vi "WritePathFile_Example.vi"(11 "Max Velocity M/S":dbl=3.2 format="%17.3f") -> (1 "PathPlannerTrajectory":T13 {"States"."TargetHolonomicRotation"."SIN" format="%13.4f"; "States"."TargetHolonomicRotation"."COS" format="%13.4f"; "States"."TargetHolonomicRotation"."VALUE" format="%13.4f"; "States"."Heading"."SIN" format="%13.4f"; "States"."Heading"."COS" format="%13.4f"; "States"."Heading"."VALUE" format="%13.4f"; "States"."PositionMeters"."Y" format="%14.3f"; "States"."PositionMeters"."X" format="%14.3f"}, 2 "Trajectory State\nCount":i32, 3 "TotalTImeSecs":dbl)   [LabVIEW 2019]
uses:
  <vilib>/Rock Robotics/WPI/ThirdParty/MJansen/PathPlanner/TypeDef/PathPlannerTrajectory.ctl
  <vilib>/Rock Robotics/WPI/ThirdParty/MJansen/PathPlanner/TypeDef/PathPlannerTrajectoryState.ctl
  <vilib>/Rock Robotics/WPI/ThirdParty/JAS_Junk/TrajLib/TypeDef/TRANSLATION2D.ctl
  <vilib>/Rock Robotics/WPI/ThirdParty/JAS_Junk/TrajLib/TypeDef/ROTATION2D.ctl
  <vilib>/Rock Robotics/WPI/ThirdParty/MJansen/PathPlanner/TypeDef/PathPlannerPathConstraints.ctl
  <vilib>/Rock Robotics/WPI/ThirdParty/MJansen/PathPlanner/TypeDef/PathPlannerPath.ctl
  <vilib>/Rock Robotics/WPI/ThirdParty/MJansen/PathPlanner/TypeDef/PathPlannerRotationTarget.ctl
  <vilib>/Rock Robotics/WPI/ThirdParty/MJansen/PathPlanner/TypeDef/PathPlannerConstraintsZone.ctl
  <vilib>/Rock Robotics/WPI/ThirdParty/MJansen/PathPlanner/TypeDef/PathPlannerEventMarker.ctl
  <vilib>/Rock Robotics/WPI/ThirdParty/MJansen/PathPlanner/TypeDef/PathPlannerCommandUtil.ctl
  <vilib>/Rock Robotics/WPI/ThirdParty/MJansen/PathPlanner/ENum/PathPlanner_CommandUtilType_ENUM.ctl
  <vilib>/Rock Robotics/WPI/ThirdParty/MJansen/PathPlanner/TypeDef/PathPlannerGoalEndState.ctl
  <vilib>/Rock Robotics/WPI/ThirdParty/MJansen/PathPlanner/TypeDef/PathPlannerPathPoint.ctl
  <vilib>/Rock Robotics/WPI/ThirdParty/JAS_Junk/TrajLib/Rotation2d_CreateAngle.vi
  <vilib>/Rock Robotics/WPI/ThirdParty/JAS_Junk/TrajLib/Translation2d_Create.vi
  <vilib>/Rock Robotics/WPI/ThirdParty/JAS_Junk/TrajLib/Pose2d_getTranslation.vi
  <vilib>/Rock Robotics/WPI/ThirdParty/JAS_Junk/TrajLib/Translation2d_GetDistance.vi
  <vilib>/Rock Robotics/WPI/ThirdParty/JAS_Junk/TrajLib/Pose2d_getRotation.vi
  <vilib>/Rock Robotics/WPI/ThirdParty/JAS_Junk/TrajLib/Translation2d_Create_DistAng.vi
  <vilib>/Rock Robotics/WPI/ThirdParty/JAS_Junk/TrajLib/Translation2d_Plus.vi
  <vilib>/Rock Robotics/WPI/ThirdParty/JAS_Junk/TrajLib/Rotation2d_Plus.vi
  <vilib>/Rock Robotics/WPI/ThirdParty/JAS_Junk/TrajLib/Util_CalcDist.vi
  <vilib>/Rock Robotics/WPI/ThirdParty/JAS_Junk/TrajLib/Rotation2d_GetAngleCosSin.vi
  <vilib>/Rock Robotics/WPI/ThirdParty/JAS_Junk/TrajLib/Rotation2d_RotateBy.vi
  <vilib>/Rock Robotics/WPI/ThirdParty/JAS_Junk/TrajLib/Rotation2d_CreateXY.vi
  <vilib>/Rock Robotics/WPI/ThirdParty/MJansen/PathPlanner/PathPlanner24.lvlib
  <vilib>/Rock Robotics/WPI/ThirdParty/JAS_Junk/TrajLib/Trajectory_Library.lvlib
panel:
  out "Write File Error":errorcluster
  in  "Write Path File":bool
  in  "Path":path
  out "PathPlannerPath":T1={"BezierPoints"=[], "PreviewStartingRotation"={"VALUE"=0.0, "COS"=1.0, "SIN"=0.0}, "Reversed"=FALSE, "RotationTargets"=[], "ConstraintZones"=[], "EventMarkers"=[], "GlobalConstraints"={"MaxVelocityMps;"=0.0, "MaxAccelerationMpsSq;"=0.0, "MaxAngularVelRadPsEc;"=0.0, "MaxAngularAccRadPSecSq"=0.0, "Exists"=FALSE}, "GoalEndState"={"Velocity"=0.0, "Rotation"={"VALUE"=0.0, "COS"=1.0, "SIN"=0.0}}, "AllPoints"=[]} {"AllPoints"."HolonomicRotation"."SIN" format="%13.4f"; "AllPoints"."HolonomicRotation"."COS" format="%13.4f"; "AllPoints"."HolonomicRotation"."VALUE" format="%13.4f"; "AllPoints"."Position"."Y" format="%14.3f"; "AllPoints"."Position"."X" format="%14.3f"; "GoalEndState"."Rotation"."SIN" format="%13.4f"; "GoalEndState"."Rotation"."COS" format="%13.4f"; "GoalEndState"."Rotation"."VALUE" format="%13.4f"; "EventMarkers"."lastRobotPos"."Y" format="%14.3f"; "EventMarkers"."lastRobotPos"."X" format="%14.3f"; "EventMarkers"."markerPos"."Y" format="%14.3f"; "EventMarkers"."markerPos"."X" format="%14.3f"; "RotationTargets"."target"."SIN" format="%13.4f"; "RotationTargets"."target"."COS" format="%13.4f"; "RotationTargets"."target"."VALUE" format="%13.4f"; "PreviewStartingRotation"."SIN" format="%13.4f"; "PreviewStartingRotation"."COS" format="%13.4f"; "PreviewStartingRotation"."VALUE" format="%13.4f"; "BezierPoints"."Y" format="%14.3f"; "BezierPoints"."X" format="%14.3f"}
  in  "End Angle Degrees":dbl format="%#_13g"
  in  "End Velocity M/S":dbl format="%#_13g"
  in  "Start Angual Vel Rad/S":dbl format="%#_13g"
  in  "Start Y Vel M/S":dbl format="%#_13g"
  in  "Start X Vel M/S":dbl format="%#_13g"
  in  "MaxAngularAccel Radians.Sec^2":dbl=2.4 format="%17.3f"
  in  "Point 4":T12={"X Meters"=3.0, "Y Meters"=3.0, "Heading  Deg"=90.0} {"Heading  Deg" format="%13.3f"; "Y Meters" format="%13.3f"; "X Meters" format="%13.3f"}
  in  "Point 3":T12={"X Meters"=3.0, "Y Meters"=2.7, "Heading  Deg"=90.0} {"Heading  Deg" format="%13.3f"; "Y Meters" format="%13.3f"; "X Meters" format="%13.3f"}
  in  "Point 2":T12={"X Meters"=1.3, "Y Meters"=1.0, "Heading  Deg"=0.0} {"Heading  Deg" format="%13.3f"; "Y Meters" format="%13.3f"; "X Meters" format="%13.3f"}
  out "Path\nCreation\nError":bool
  out "Trajectory":cluster{dbl[], dbl[]}(graph)
  in  "Initial Point":T12={"X Meters"=1.0, "Y Meters"=1.0, "Heading  Deg"=0.0} {"Heading  Deg" format="%13.3f"; "Y Meters" format="%13.3f"; "X Meters" format="%13.3f"}
  in  "MaxAcceleration M/S^2":dbl=2.8 format="%17.1f"
  in  "MaxAngularVel  Radians/Sec":dbl=1.8 format="%17.3f"
  # "Create PathPlanner Path/Trajectory Sample"
  # "This VI is designed to be called by BEGIN.VI, but can be executed directly to test trajectory parameters."
  # "CREATED TRAJECTORY INFORMATION"
  # "PATH CONFIGURATION"
  # "PATH DEFINITION"
  # "There can be as many points as needed."
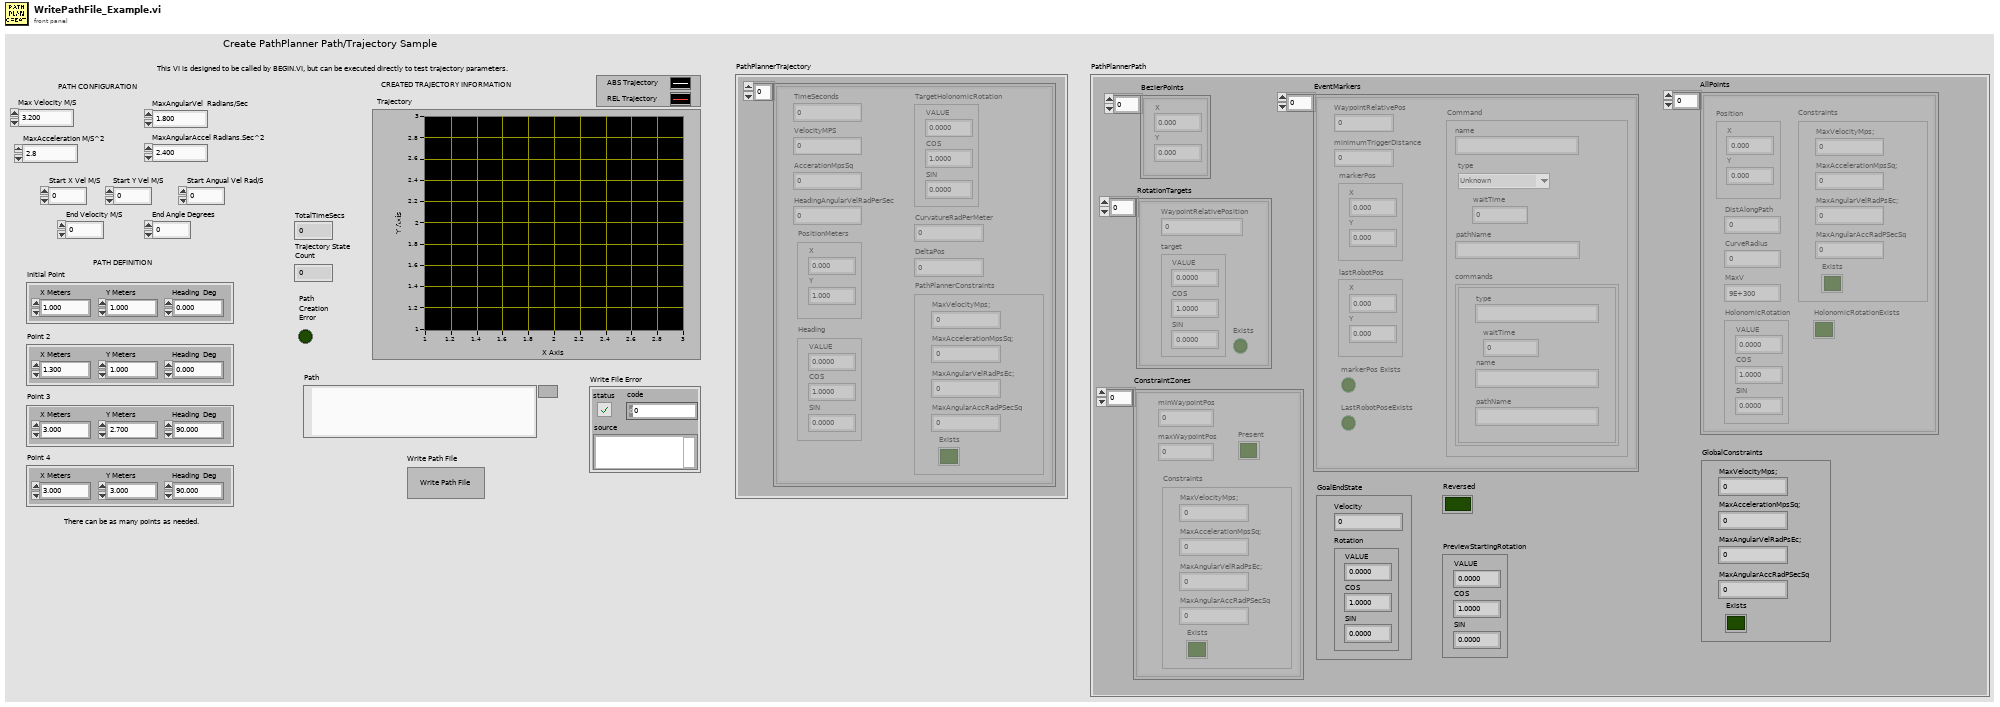
[diagram p1: front panel]
types:
  T1 = typedef "PathPlanner24.lvlib/PathPlannerPath.ctl" = cluster{"BezierPoints":T2[], "PreviewStartingRotation":T3, "Reversed":bool, "RotationTargets":T4[], "ConstraintZones":T5[], "EventMarkers":T7[], "GlobalConstraints":T6, "GoalEndState":T10, "AllPoints":T11[]}
  T2 = typedef "Trajectory_Library.lvlib/TRANSLATION2D.ctl" = cluster{"X":dbl, "Y":dbl}
  T3 = typedef "Trajectory_Library.lvlib/ROTATION2D.ctl" = cluster{"VALUE":dbl, "COS":dbl, "SIN":dbl}
  T4 = typedef "PathPlanner24.lvlib/PathPlannerRotationTarget.ctl" = cluster{"target":T3, "WaypointRelativePosition":dbl, "Exists":bool}
  T5 = typedef "PathPlanner24.lvlib/PathPlannerConstraintsZone.ctl" = cluster{"minWaypointPos":dbl, "maxWaypointPos":dbl, "Constraints":T6, "Present":bool}
  T6 = typedef "PathPlanner24.lvlib/PathPlannerPathConstraints.ctl" = cluster{"MaxVelocityMps;":dbl, "MaxAccelerationMpsSq;":dbl, "MaxAngularVelRadPsEc;":dbl, "MaxAngularAccRadPSecSq":dbl, "Exists":bool}
  T7 = typedef "PathPlanner24.lvlib/PathPlannerEventMarker.ctl" = cluster{"WaypointRelativePos":dbl, "minimumTriggerDistance":dbl, "markerPos":T2, "lastRobotPos":T2, "Command":T8, "markerPos Exists":bool, "LastRobotPoseExists":bool}
  T8 = typedef "PathPlanner24.lvlib/PathPlannerCommandUtil.ctl" = cluster{"waitTime":dbl, "name":string, "pathName":string, "commands":cluster{"type":string, "waitTime":dbl, "name":string, "pathName":string}[], "type":T9}
  T9 = typedef "PathPlanner24.lvlib/PathPlanner_CommandUtilType_ENUM.ctl" = enum16{"Unknown", "Wait", "Named", "Path", "Sequential", "Parallel", "Race", "Deadline"}
  T10 = typedef "PathPlanner24.lvlib/PathPlannerGoalEndState.ctl" = cluster{"Velocity":dbl, "Rotation":T3}
  T11 = typedef "PathPlanner24.lvlib/PathPlannerPathPoint.ctl" = cluster{"Position":T2, "HolonomicRotation":T3, "DistAlongPath":dbl, "CurveRadius":dbl, "MaxV":dbl, "Constraints":T6, "HolonomicRotationExists":bool}
  T12 = cluster{"X Meters":dbl, "Y Meters":dbl, "Heading  Deg":dbl}
  T13 = typedef "PathPlanner24.lvlib/PathPlannerTrajectory.ctl" = cluster{"States":T14[]}
  T14 = typedef "PathPlanner24.lvlib/PathPlannerTrajectoryState.ctl" = cluster{"TimeSeconds":dbl, "VelocityMPS":dbl, "AccerationMpsSq":dbl, "HeadingAngularVelRadPerSec":dbl, "PositionMeters":T2, "Heading":T3, "TargetHolonomicRotation":T3, "CurvatureRadPerMeter":dbl, "PathPlannerConstraints":T6, "DeltaPos":dbl}
  T15 = typedef "Trajectory_Library.lvlib/POSE2D.ctl" = cluster{"TRANSLATION":T2, "ROTATION":T3}
  T16 = typedef "Trajectory_Library.lvlib/CHASSIS_SPEEDS.ctl" = cluster{"vX":dbl, "vY":dbl, "vOmega":dbl}
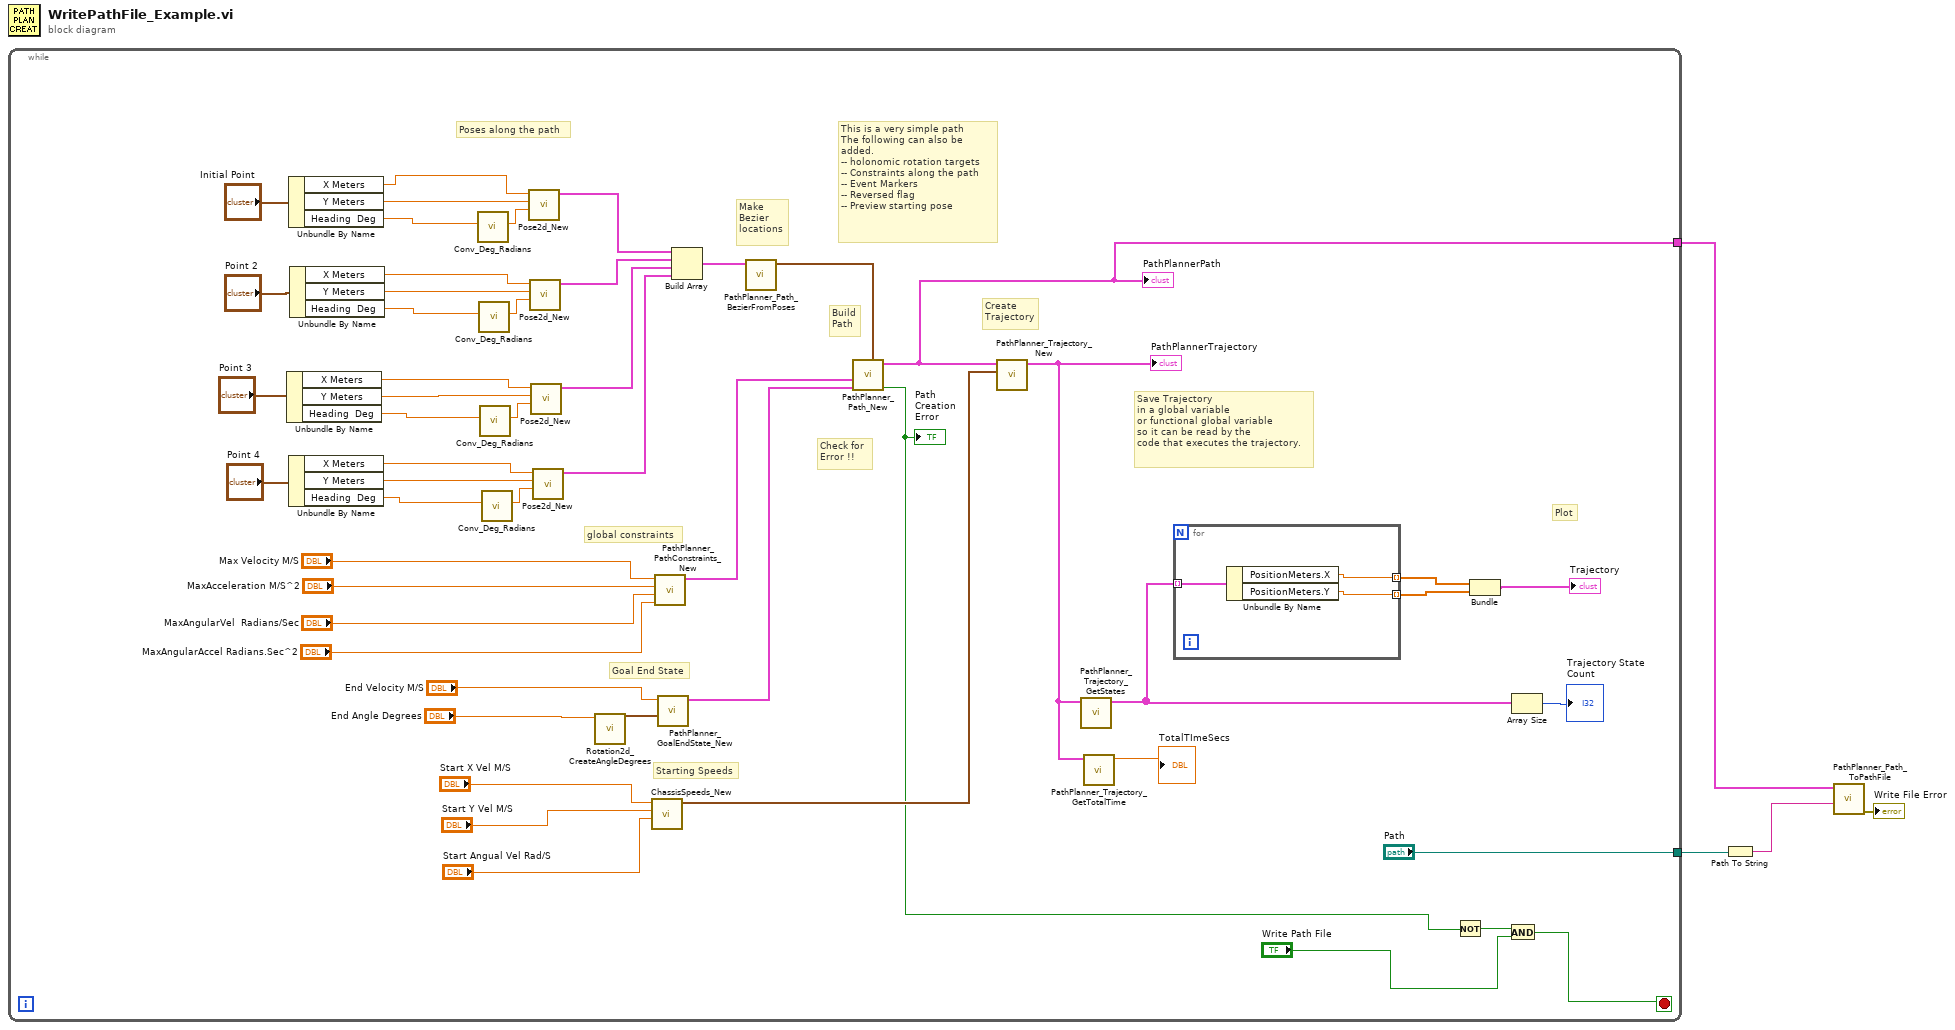
[diagram p0: block diagram]
diagram:
  n1 = while {
    tunnel: ["Path"] -> w4
    tunnel: [w6] -> w2
    stop <- w8 stop-if-true
    # "This is a very simple path\nThe following can also be\nadded.\n-- holonomic rotation targets\n-- Constraints along the path\n-- Event Markers\n-- Reversed flag\n-- Preview starting pose"
    # "Plot"
    # "Save Trajectory\nin a global variable\nor functional global variable\nso it can be read by the \ncode that executes the trajectory."
    # "Create\nTrajectory"
    # "Check for\nError !!"
    # "Starting Speeds"
    # "Goal End State"
    # "global constraints"
    # "Make\nBezier\nlocations"
    # "Build\nPath"
    # "Poses along the path"
    n2 = Unbundle By Name("Point 3") -> ("X Meters"=w20:dbl, "Y Meters"=w19:dbl, "Heading  Deg"=w18:dbl)
    n3 = Unbundle By Name("Initial Point") -> ("X Meters"=w28:dbl, "Y Meters"=w27:dbl, "Heading  Deg"=w26:dbl)
    n4 = Unbundle By Name("Point 4") -> ("X Meters"=w17:dbl, "Y Meters"=w16:dbl, "Heading  Deg"=w15:dbl)
    n5 = Unbundle By Name("Point 2") -> ("X Meters"=w25:dbl, "Y Meters"=w24:dbl, "Heading  Deg"=w23:dbl)
    n6 = call <vilib>:"Conv_Deg_Radians.vi"("Degress"=w26) -> ("Radians"=w38:dbl)  [unwired: 10 in]
    n7 = call <vilib>:"Conv_Deg_Radians.vi"("Degress"=w23) -> ("Radians"=w39:dbl)  [unwired: 10 in]
    n8 = call <vilib>:"Conv_Deg_Radians.vi"("Degress"=w18) -> ("Radians"=w40:dbl)  [unwired: 10 in]
    n9 = call <vilib>:"Conv_Deg_Radians.vi"("Degress"=w15) -> ("Radians"=w41:dbl)  [unwired: 10 in]
    n10 = call <vilib>:"Pose2d_New.vi"("Heading"=w38, "Y"=w27, "X"=w28) -> ("out POSe"=w42:T15)  [unwired: 8 in]
    n11 = call <vilib>:"Pose2d_New.vi"("Heading"=w39, "Y"=w24, "X"=w25) -> ("out POSe"=w43:T15)  [unwired: 8 in]
    n12 = call <vilib>:"Pose2d_New.vi"("Heading"=w40, "Y"=w19, "X"=w20) -> ("out POSe"=w44:T15)  [unwired: 8 in]
    n13 = call <vilib>:"Pose2d_New.vi"("Heading"=w41, "Y"=w16, "X"=w17) -> ("out POSe"=w45:T15)  [unwired: 8 in]
    n14 = call <vilib>:"Rotation2d_CreateAngleDegrees.vi"("Angle_Degrees"="End Angle Degrees") -> ("ROTATION"=w49:T3)  [unwired: 10 in]
    n15 = call <vilib>:"ChassisSpeeds_New.vi"("vAngular"="Start Angual Vel Rad/S", "vY"="Start Y Vel M/S", "vX"="Start X Vel M/S") -> ("CHASSIS"=w55:T16)  [unwired: 8 in]
    n16 = call <vilib>:"PathPlanner_PathConstraints_New.vi"("MaxAngularAccRadPSecSq"="MaxAngularAccel Radians.Sec^2", "MaxAngularVelRadPsEc;"="MaxAngularVel  Radians/Sec", "MaxAccelerationMpsSq;"="MaxAcceleration M/S^2", "MaxVelocityMps;"="Max Velocity M/S") -> ("PathPlannerConstraints"=w47:T6)  [unwired: 7 in]
    n17 = call <vilib>:"PathPlanner_GoalEndState_New.vi"("Rotation"=w49, "Velocity"="End Velocity M/S") -> ("GoalEndState"=w51:T10)  [unwired: 9 in]
    n18 = Build Array(w42, w43, w44, w45) -> (w37:T15[])
    n19 = call <vilib>:"PathPlanner_Path_BezierFromPoses.vi"("Poses"=w37) -> ("Bezier"=w46:T2[])  [unwired: 9 in, 1 out]
    n20 = call <vilib>:"PathPlanner_Path_New.vi"("BezierPoints"=w46, "GoalEndState"=w51, "GlobalConstraints"=w47) -> ("Error"=w5:bool, "PathPlannerPath"=w6:T1)  [unwired: 7 in]
    "Path\nCreation\nError" <- w5
    "PathPlannerPath" <- w6
    n21 = call <vilib>:"PathPlanner_Trajectory_New.vi"("StartingSpeeds"=w55, "Path"=w6) -> ("PathPlannerTrajectory"=w32:T13)  [unwired: 9 in]
    "PathPlannerTrajectory" <- w32
    n22 = call <vilib>:"PathPlanner_Trajectory_GetStates.vi"("PathPlannerTrajectory"=w32) -> ("PathPlannerStates"=w33:T14[])  [unwired: 10 in]
    n23 = call <vilib>:"PathPlanner_Trajectory_GetTotalTime.vi"("PathPlannerTrajectory"=w32) -> ("TotalTimeSeconds"=→"TotalTImeSecs":dbl)  [unwired: 10 in]
    n24 = for {
      tunnel: [w59] -> w35 mode=indexing
      tunnel: [w58] -> w36 mode=indexing
      tunnel: w33 -> [w57] mode=indexing
      n25 = Unbundle By Name(w57) -> ("PositionMeters.X"=w59:dbl, "PositionMeters.Y"=w58:dbl)
    }
    n26 = Not(x=w5) -> (.not. x?=w10:bool)
    n27 = Bundle(w35, w36) -> (→"Trajectory":cluster{dbl[], dbl[]})  [unwired: 1 in]
    n28 = And(x=w10, y="Write Path File") -> (x .and. y?=w8:bool)
    n29 = Array Size(array=w33) -> (size(s)=→"Trajectory State\nCount":i32)
  }
  n30 = Path To String(path=w4) -> (string=w3:string)
  n31 = call <vilib>:"PathPlanner_Path_ToPathFile.vi"("FileName"=w3, "PathPlannerPath"=w2) -> ("error out"=→"Write File Error":errorcluster)  [unwired: 8 in, 1 out]
